vi "New Results (to override).vi"(7 "Image Nr.":i32, 8 "error in (no error)":errorcluster, 9 "Results In":refnum<class "Analyze Results Base.lvclass">[](array[class]), 10 "Parameters":refnum<class "Analyze Parameter Base.lvclass">[](array[class]), 11 "HIJ Single Cam App Demo In":refnum<class "HIJ Single Cam App Demo.lvclass">) -> (0 "error out":errorcluster, 3 "HIJ Single Cam App Demo Out":refnum<class "HIJ Single Cam App Demo.lvclass">)   [LabVIEW 2014, in "HIJ Single Cam App Demo.lvlib" / "HIJ Single Cam App Demo.lvclass"]
uses:
  HIJ Single Cam App Demo.lvclass
  Analyze/Results and Overlays/Results Base/Analyze Results Base.lvclass
  Analyze/Analyze Parameter/Analyze Parameter Base/Analyze Parameter Base.lvclass
  <vilib>/ActorFramework/Actor/Actor.lvclass/Actor.ctl
  HIJ Single Cam App Demo.lvclass/HIJ Single Cam App Demo.ctl
  Abstract Messages/Publish Analyze Results Msg/Publish Analyze Results Msg.lvclass/Publish Analyze Results Msg.ctl
  <vilib>/ActorFramework/Message Enqueuer/Message Enqueuer.lvclass/Message Enqueuer.ctl
  <vilib>/ActorFramework/Message Enqueuer/Enqueue.vi
  <vilib>/ActorFramework/Message Priority Queue/Priority Enqueue.vi
  HIJ Vision Camera App/HIJ Vision Camera App/HIJ Vision Camera App.lvclass
  <vilib>/ActorFramework/Message Enqueuer/Message Enqueuer.lvclass
  <vilib>/ActorFramework/Actor/Actor.lvclass
  Abstract Messages/Publish Analyze Results Msg/Publish Analyze Results Msg.lvclass
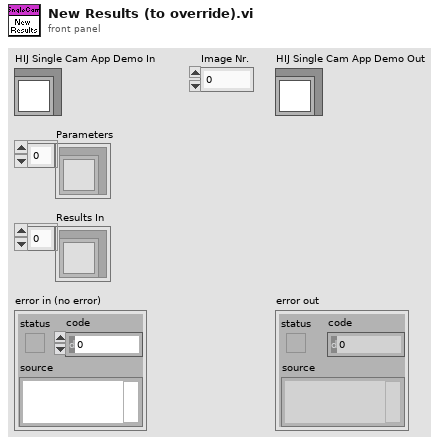
[diagram p1: front panel]
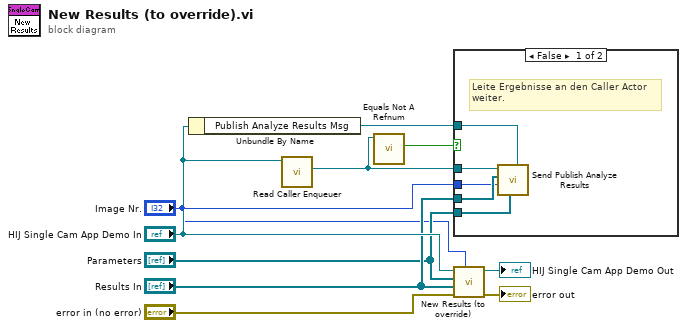
[diagram p0: block diagram]
diagram:
  n1 = Unbundle By Name("HIJ Single Cam App Demo In") -> ("Publish Analyze Results Msg"=w6:refnum<class "Publish Analyze Results Msg.lvclass">)
  n2 = call <vilib>:"Read Caller Enqueuer.vi"("Actor"="HIJ Single Cam App Demo In") -> ("Caller Enqueuer"=w3:refnum<class "Message Enqueuer.lvclass">)  [unwired: 10 in]
  n3 = call <vilib>:"Equals Not A Refnum.vi"("Message Enqueuer"=w3) -> ("Not a refnum?"=w2:bool)  [unwired: 10 in]
  n4 = case shown="False" w2 {
    tunnel: w6 -> [w15 _]
    tunnel: "Results In" -> [w14 _]
    tunnel: "Parameters" -> [w13 _]
    tunnel: w3 -> [w12 _]
    tunnel: "Image Nr." -> [w11 _]
    frame False {
      # "Leite Ergebnisse an den Caller Actor\nweiter."
      n5 = call "Send Publish Analyze Results.vi"("Message Type"=w15, "Parameters"=w13, "Image Nr."=w11, "Results In"=w14, "Message Enqueuer"=w12) -> ()  [unwired: 5 in, 2 out]
    }
    frame True {
    }
  }
  n6 = call-parent "New Results (to override).vi"("Image Nr."="Image Nr.", "error in (no error)"="error in (no error)", "Results In"="Results In", "Parameters"="Parameters", "HIJ Vision Camera App In"="HIJ Single Cam App Demo In") -> ("error out"=→"error out":errorcluster, "HIJ Vision Camera App Out"=→"HIJ Single Cam App Demo Out":refnum<class "HIJ Single Cam App Demo.lvclass">)  [unwired: 5 in]
